vi "Start Up Options.vi"(1 "Error In":errorcluster) -> (0 "Error Out":errorcluster)   [LabVIEW 2018]
uses:
  Type Defs/RT Startup options.ctl
  Type Defs/RT Command.ctl
panel:
  in  "Source Exhaust Low":bool=TRUE
  out "All On":bool
  in  "Out of Gas Flag":bool=TRUE
  in  "System Polling":bool=TRUE
  in  "Turbo Speed":bool=TRUE
  in  "Foreline Pressure":bool=TRUE
  in  "Drying Gas":bool=TRUE
  in  "Door Interlock":bool=TRUE
  in  "Done":bool
  # "For turning on and off the interloack checking sequence during start up."
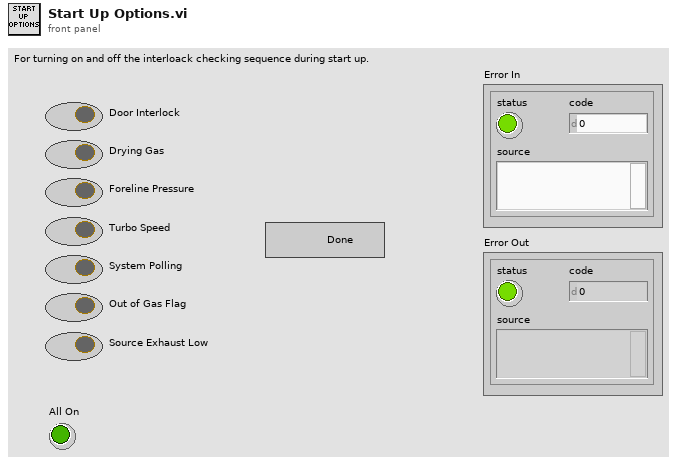
[diagram p1: front panel]
types:
  T1 = typedef "RT Command.ctl" = enum16{"xml Start Run", "xml Start Actual Run", "xml Stop Run", "xml Runtime Update", "xml Get Status", "xml Get Table", "xml Set Table", "xml Get Configuration", "xml System Status", "xml Set LC Input Logic", "xml Get Data", "xml Get Info", "Start", "StartActualRun", "Stop", "Runtime Update", "Get Data", "Get Info", "Get Status", "Get Param", "Get Config", "Get Table", "Read ADC", "Set Oscillator", "Update Config", "Update Table", "Set All Pol", "Set Pol and DC", "Set Max Mass", "Toggle RP", "Toggle EL", "Set PIC", "Initialize Turbo", "Send Turbo Comm", "Close Turbo", "P1", "P2", "P3", "Send Serial", "Set LC Out", "Get LC In", "Read VAC", "Test Table", "Toggle Power", "Get Startup", "Set Startup", "Get ADC Table", "Set ADC Table", "Get Brief Status", "Get Detail Status", "Auxiliary Update", "Set CC Logics", "Set CC Input Logics", "Ignore Error", "invalid"}
  T2 = typedef "RT Startup options.ctl" = cluster{"Door":bool, "Curtain":bool, "Pressure":bool, "Turbo":bool, "SysPoll":bool, "GasFlag":bool, "SourceExhaust":bool}
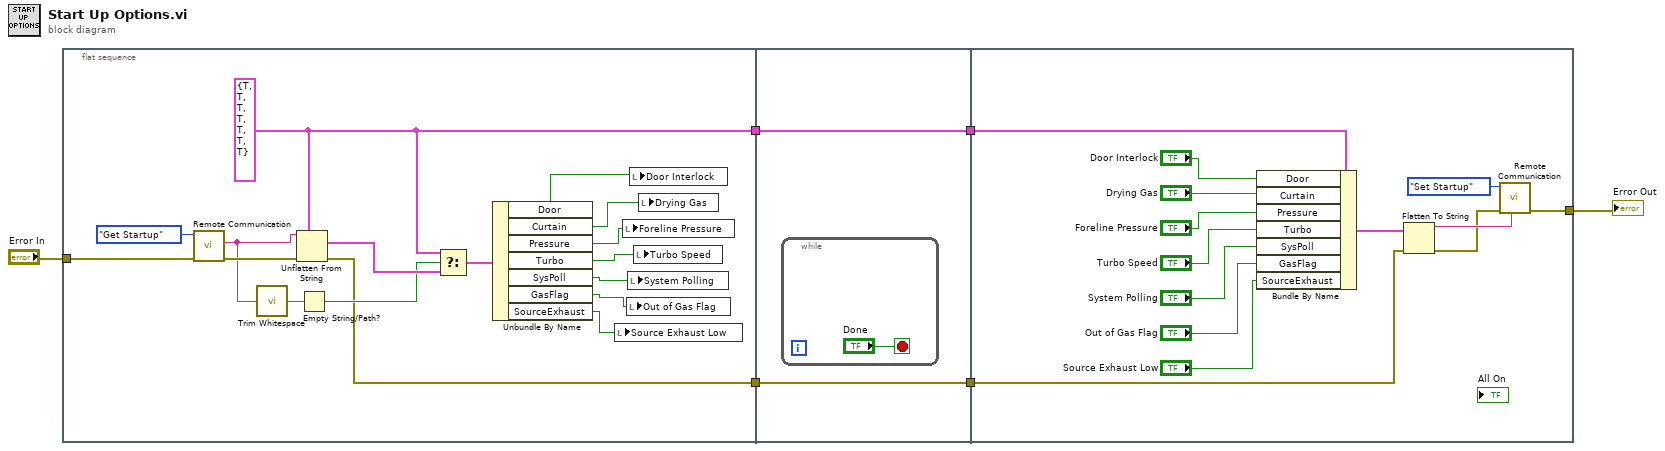
[diagram p0: block diagram]
diagram:
  n1 = flat-sequence {
    tunnel: "Error In" -> [w17]
    tunnel: [w9] -> w5
    tunnel: [w7] -> w2
    tunnel: w5 -> [w25]
    tunnel: [w25] -> w4
    tunnel: [w24] -> w3
    tunnel: w2 -> [w24]
    tunnel: w4 -> [w31]
    tunnel: w3 -> [w40]
    tunnel: [w28] -> w1
    frame #0 {
      w7 = T2 {"Door"=TRUE, "Curtain"=TRUE, "Pressure"=TRUE, "Turbo"=TRUE, "SysPoll"=TRUE, "GasFlag"=TRUE, "SourceExhaust"=TRUE} ("StartupOptions")
      n2 = call "Remote Communication.vi"("Error In"=w17, "Command"=RT_Command."Get Startup") -> ("Error Out"=w19:errorcluster, "Info"=w8:string)  [unwired: 4 in, 2 out]
      n3 = call <vilib>:"Trim Whitespace.vi"("string"=w8) -> ("trimmed string"=w22:string)  [unwired: 1 in]
      n4 = Unflatten From String(type=w7, binary string=w8, error in (no error)=w19) -> (value=w21:T2, error out=w9:errorcluster)  [unwired: 3 out]
      n5 = Empty String/Path?(string/path=w22) -> (empty?=w20:bool)
      n6 = Select(t=w7, s=w20, f=w21) -> (s? t:f=w18:T2)
      n7 = Unbundle By Name(w18) -> ("Door"=w16:bool, "Curtain"=w15:bool, "Pressure"=w14:bool, "Turbo"=w13:bool, "SysPoll"=w12:bool, "GasFlag"=w11:bool, "SourceExhaust"=w10:bool)
      n8 = local write "Source Exhaust Low"(w10) -> ()
      n9 = local write "Foreline Pressure"(w14) -> ()
      n10 = local write "Out of Gas Flag"(w11) -> ()
      n11 = local write "System Polling"(w12) -> ()
      n12 = local write "Door Interlock"(w16) -> ()
      n13 = local write "Turbo Speed"(w13) -> ()
      n14 = local write "Drying Gas"(w15) -> ()
    }
    frame #1 {
      n15 = while {
        stop <- "Done" stop-if-true
      }
    }
    frame #2 {
      n16 = Bundle By Name(cluster=w40, "Door"="Door Interlock", "Curtain"="Drying Gas", "Pressure"="Foreline Pressure", "Turbo"="Turbo Speed", "SysPoll"="System Polling", "GasFlag"="Out of Gas Flag", "SourceExhaust"="Source Exhaust Low") -> (w32:T2)
      n17 = Flatten To String(anything=w32, error in (no error)=w31) -> (data string=w30:string, error out=w29:errorcluster)  [unwired: 3 out]
      n18 = call "Remote Communication.vi"("String"=w30, "Error In"=w29, "Command"=RT_Command."Set Startup") -> ("Error Out"=w28:errorcluster)  [unwired: 3 in, 3 out]
    }
  }
  "Error Out" <- w1
